vi "MGI Get Listbox String[][].vi"(11 "MGI Error Dialog in":refnum<class "MGI Error Reporter Dialog.lvclass">) -> (1 "Error[Row][Err/Warn,Name,Time,Count]":string[][](array[string]), 3 "MGI Error Dialog out":refnum<class "MGI Error Reporter Dialog.lvclass">)   [LabVIEW 2016, in "MGI Error Reporter Dialog.lvclass"]
doc: "Output all processed errors that have not been cleared by the user as a 2D array of strings. There is a row for each error, and the columns for a row are:\nColumn 0: \"Err\" for an error and \"Warn\" for warning\nColumn 1: A short name representing the error code. For code 1, this string is \"Argument Error\"\nColumn 2: The time and date the error was processed.\nColumn 3: The count of how many times this error has occurred in the current run or since this error was last cleared.\n\nAuthored by Shawn Walpole\nsupport@mooregoodideas.com\nwww.mooregoodideas.com\n\nCopyright (c) 2013, Moore Good Ideas, Inc.\n\nAll rights reserved.\n\nRedistribution and use in source and binary forms, with or without modification, are permitted provided that the following conditions are met:\n\n * Redistributions of source code must retain the above copyright notice, this list of conditions and the following disclaimer.\n * Redistributions in binary form must reproduce the above copyright notice, this list of conditions and the following disclaimer in the documentation and/or other materials provided with the distribution.\n * Neither the name of Moore Good Ideas, Inc. nor the names of its contributors may be used to endorse or promote products derived from this software without specific prior written permission.\n\nTHIS SOFTWARE IS PROVIDED BY THE COPYRIGHT HOLDERS AND CONTRIBUTORS \"AS IS\" AND ANY EXPRESS OR IMPLIED WARRANTIES, INCLUDING, BUT NOT LIMITED TO, THE IMPLIED WARRANTIES OF MERCHANTABILITY AND FITNESS FOR A PARTICULAR PURPOSE ARE DISCLAIMED. IN NO EVENT SHALL THE COPYRIGHT OWNER OR CONTRIBUTORS BE LIABLE FOR ANY DIRECT, INDIRECT, INCIDENTAL, SPECIAL, EXEMPLARY, OR CONSEQUENTIAL DAMAGES (INCLUDING, BUT NOT LIMITED TO, PROCUREMENT OF SUBSTITUTE GOODS OR SERVICES; LOSS OF USE, DATA, OR PROFITS; OR BUSINESS INTERRUPTION) HOWEVER CAUSED AND ON ANY THEORY OF LIABILITY, WHETHER IN CONTRACT, STRICT LIABILITY, OR TORT (INCLUDING NEGLIGENCE OR OTHERWISE) ARISING IN ANY WAY OUT OF THE USE OF THIS SOFTWARE, EVEN IF ADVISED OF THE POSSIBILITY OF SUCH DAMAGE."
uses:
  <userlib>/_MGI/Error Reporter/MGI Error Reporter Dialog/MGI Error Reporter Dialog.lvclass
  C:/Program Files (x86)/National Instruments/LabVIEW 2016/user.lib/_MGI/Error Reporter/MGI Error Reporter Base/MGI Error Reporter Base.lvclass
  <userlib>/_MGI/Error Reporter/MGI Error Reporter Dialog/MGI Error Reporter Dialog.lvclass/MGI Error Reporter Dialog.ctl
  <userlib>/_MGI/Error Reporter/MGI Error Reporter Dialog/MGI ERD LB Row Base/MGI ERD LB Row Base.lvclass
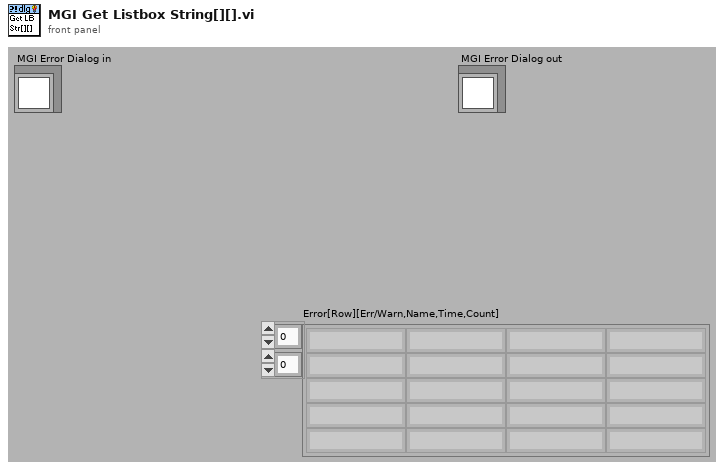
[diagram p1: front panel]
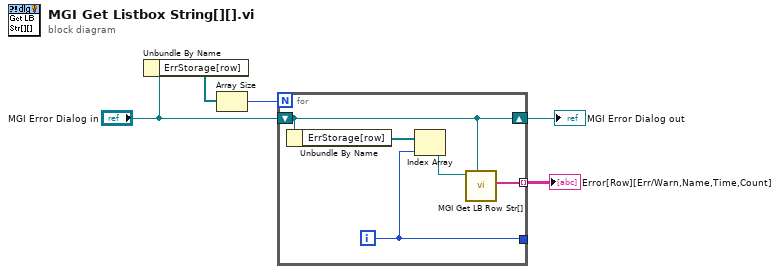
[diagram p0: block diagram]
diagram:
  n1 = Unbundle By Name("MGI Error Dialog in") -> ("ErrStorage[row]"=w1:refnum<class "MGI ERD LB Row Base.lvclass">[])
  n2 = Array Size(array=w1) -> (size(s)=w2:i32)
  n3 = for {
    N: w2 -> [_]
    tunnel: [w10] -> w5 mode=indexing
    tunnel: [w6] -> _
    shift-right: [w9] -> w4
    shift-left: "MGI Error Dialog in" -> [w9]
    i -> [w6]
    n4 = Unbundle By Name(w9) -> ("ErrStorage[row]"=w8:refnum<class "MGI ERD LB Row Base.lvclass">[])
    n5 = Index Array(array=w8, index=w6) -> (element=w7:refnum<class "MGI ERD LB Row Base.lvclass">)
    n6 = call-dynamic "MGI Get LB Row Str[].vi"("MGI Error Reporter Base In"=w9, "MGI ERD LB Row Base in"=w7) -> ("String[col]"=w10:string[])  [unwired: 2 in, 7 out]
  }
  "MGI Error Dialog out" <- w4
  "Error[Row][Err/Warn,Name,Time,Count]" <- w5
